vi "5_23_Fxp_addation.vi"(1 "y":fxp<+/-,23,5>, 2 "x":fxp<+/-,23,5>) -> (0 "x+y":fxp<+/-,24,6> format="%.41g")   [LabVIEW 2020]
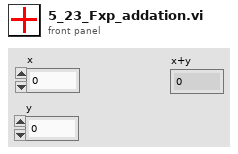
[diagram p1: front panel]
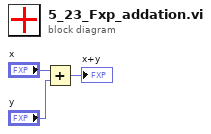
[diagram p0: block diagram]
diagram:
  n1 = Add(x="x", y="y") -> (x+y=→"x+y":fxp<+/-,24,6>)
